vi "unregisterUserEvents.vi"(8 "error in (no error)":errorcluster, 11 "tcpServer in":refnum<class "TcpServer.lvclass">) -> (0 "error out":errorcluster, 3 "tcpServer out":refnum<class "TcpServer.lvclass">)   [LabVIEW 2018, in "TcpServer.lvclass"]
doc: "Unregister User Events."
uses:
  TcpServer.lvclass
  TcpServer.lvclass/TcpServer.ctl
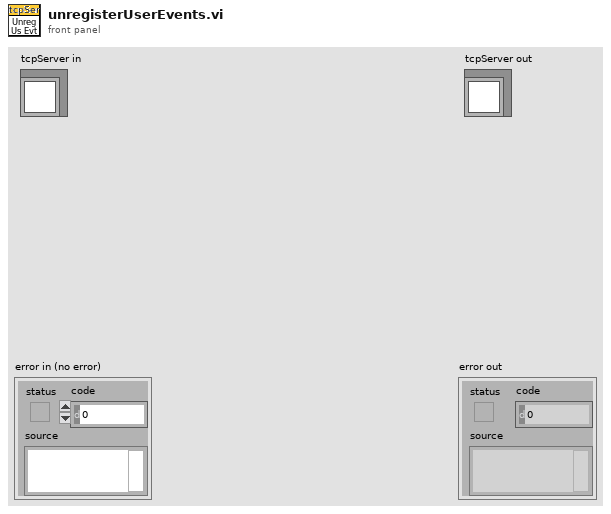
[diagram p1: front panel]
types:
  T1 = typedef "TcpServer.lvclass/userEventsTypeDef.ctl" = cluster{"TcpServer":refnum<user-event>, "Cmd":refnum<user-event>, "CmdStatus":refnum<user-event>, "Event":refnum<user-event>}
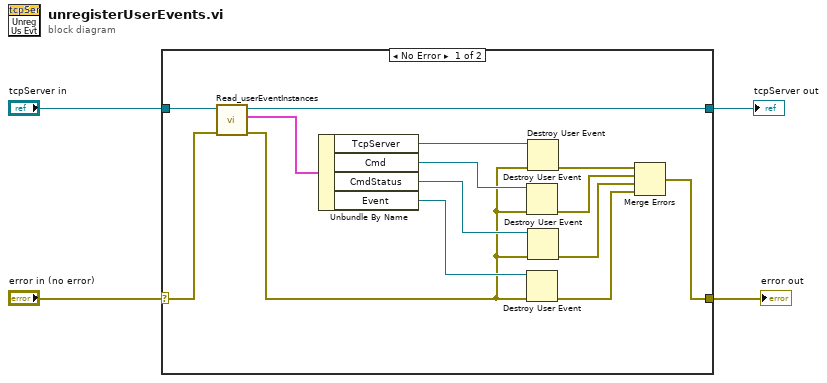
[diagram p0: block diagram]
diagram:
  n1 = case shown="No Error" "error in (no error)" {
    selector: "error in (no error)" -> [w16 w20]
    tunnel: [w12 w20] -> w3
    tunnel: [w17 w19] -> w1
    tunnel: "tcpServer in" -> [w18 w19]
    frame No Error {
      n2 = call "Read_userEventInstances.vi"("error in (no error)"=w16, "tcpServer in"=w18) -> ("error out"=w5:errorcluster, "UserEvents"=w14:T1, "tcpServer out"=w17:refnum<class "TcpServer.lvclass">)  [unwired: 7 in]
      n3 = Unbundle By Name(w14) -> ("TcpServer"=w13:refnum<user-event>, "Cmd"=w10:refnum<user-event>, "CmdStatus"=w9:refnum<user-event>, "Event"=w8:refnum<user-event>)
      n4 = Destroy User Event(user event=w10, error in=w5) -> (error out=w11:errorcluster)
      n5 = Destroy User Event(user event=w8, error in=w5) -> (error out=w6:errorcluster)
      n6 = Destroy User Event(user event=w13, error in=w5) -> (error out=w15:errorcluster)
      n7 = Destroy User Event(user event=w9, error in=w5) -> (error out=w7:errorcluster)
      n8 = Merge Errors(w15, w11, w7, w6) -> (w12:errorcluster)
    }
    frame Error {
    }
  }
  "error out" <- w3
  "tcpServer out" <- w1
